vi "AC Signal Sign.vi"(1 "Array":dbl[](array[numeric])) -> (0 "Sign1":i8)   [LabVIEW 2020]
uses:
  <vilib>/Analysis/baseanly.llb/Unimode.vi
  <vilib>/Analysis/NI_AALBase.lvlib
panel:
  out "x*y":dbl[](array[numeric])
  out "x-1":dbl[](array[numeric])
  out "0, 1":i16[](array[numeric])
  out "x > 0?":bool[](array[boolean])
  out "cos(x)":dbl[](array[numeric])
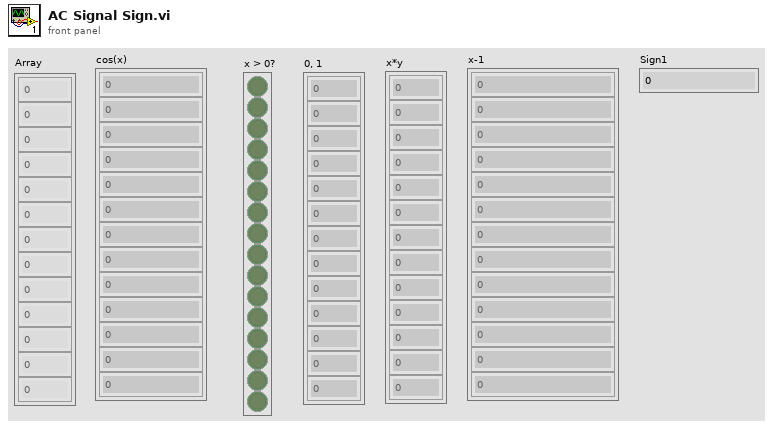
[diagram p1: front panel]
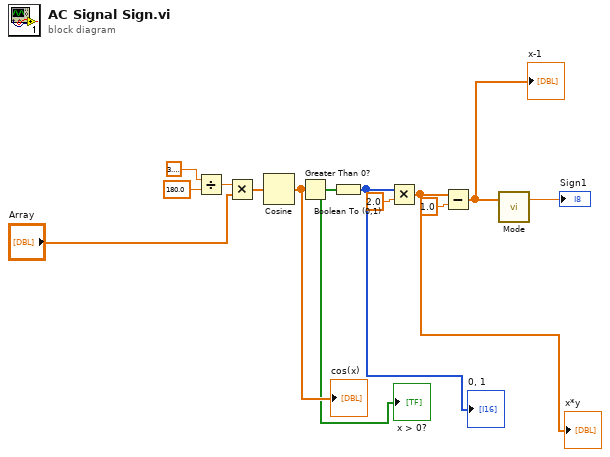
[diagram p0: block diagram]
diagram:
  n1 = Divide(x=3.141592653589793, y=180.0) -> (x/y=w7:dbl)
  n2 = Multiply(x=w7, y="Array") -> (x*y=w5:dbl[])
  n3 = Cosine(x=w5) -> (cos(x)=w13:dbl[])
  "cos(x)" <- w13
  n4 = Greater Than 0?(x=w13) -> (x > 0?=w12:bool[])
  "x > 0?" <- w12
  n5 = Boolean To (0,1)(Boolean=w12) -> (0, 1=w11:i16[])
  "0, 1" <- w11
  n6 = Multiply(x=w11, y=2.0) -> (x*y=w3:dbl[])
  "x*y" <- w3
  n7 = Subtract(x=w3, y=1.0) -> (x-y=w1:dbl[])
  "x-1" <- w1
  n8 = call-poly <vilib>:"Mode.vi"("X"=w1) -> ("mode"=→"Sign1":dbl)  [unwired: 1 in, 1 out]
